vi "Process Projects.vi"(7 "Total Memory":T1, 8 "error in (no error)":errorcluster {"code" format="Error %.0f"}, 10 "Projects":refnum<class "Project Documentation.lvclass">[](array[class]), 11 "VIDoc Printer In":refnum<class "VIDoc Printer.lvclass">) -> (0 "error out":errorcluster {"code" format="Error %.0f"}, 3 "VIDoc Printer Out":refnum<class "VIDoc Printer.lvclass">)   [LabVIEW 2023, in "VIDoc Printer.lvlib" / "VIDoc Printer.lvclass"]
uses:
  VIDoc Printer.lvclass
  <vilib>/DMC/VIDoc/Framework/UI Interaction/Interface/UI Interaction.lvclass
  Parsing/Project Documentation/Project Documentation.lvclass
  Parsing/TypeDefs/Memory Size Cluster.ctl
  Parsing/VIDoc Parsing.lvlib
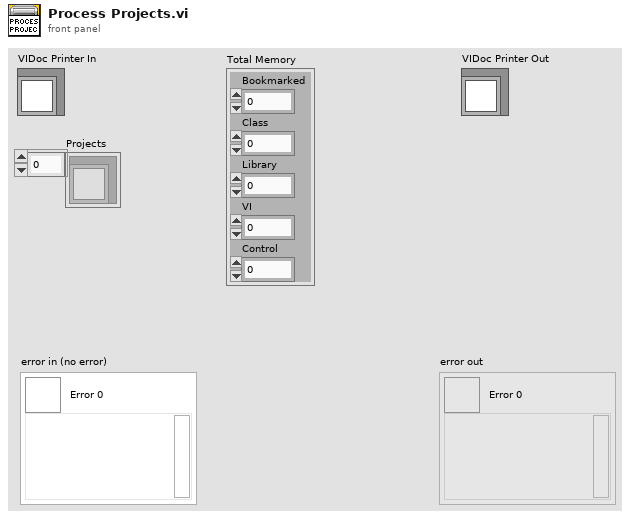
[diagram p1: front panel]
types:
  T1 = typedef "VIDoc Parsing.lvlib/Memory Size Cluster.ctl" = cluster{"Bookmarked":dbl, "Class":dbl, "Library":dbl, "VI":dbl, "Control":dbl}
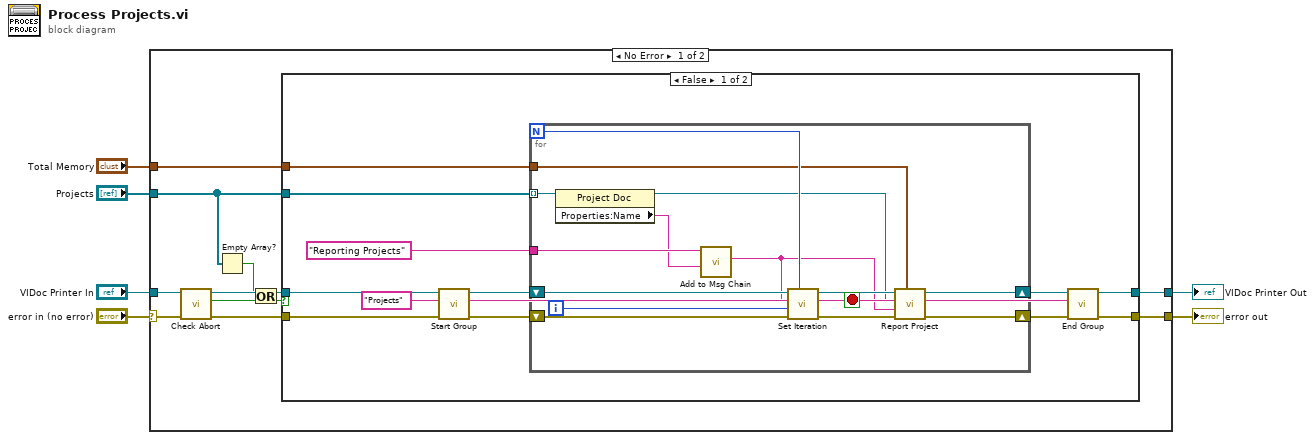
[diagram p0: block diagram]
diagram:
  n1 = case shown="No Error" "error in (no error)" {
    selector: "error in (no error)" -> [w17 w48]
    tunnel: [w12 w48] -> w5
    tunnel: [w11 w47] -> w3
    tunnel: "VIDoc Printer In" -> [w14 w47]
    tunnel: "Projects" -> [w9 _]
    tunnel: "Total Memory" -> [w10 _]
    frame No Error {
      n2 = call "Check Abort.vi"("error in (no error)"=w17, "VIDoc Printer In"=w14) -> ("error out"=w16:errorcluster, "Abort?"=w13:bool, "VIDoc Printer Out"=w15:refnum<class "VIDoc Printer.lvclass">)  [unwired: 7 in]
      n3 = Empty Array?(array=w9) -> (empty?=w7:bool)
      n4 = Or(x=w7, y=w13) -> (x .or. y?=w8:bool)
      n5 = case shown="False" w8 {
        tunnel: w9 -> [w27 _]
        tunnel: w16 -> [w26 w46]
        tunnel: w15 -> [w25 w45]
        tunnel: [w21 w46] -> w12
        tunnel: [w23 w45] -> w11
        tunnel: w10 -> [w19 _]
        frame False {
          w18 = "Projects" ("Section")
          n6 = call-dynamic "Start Group.vi"("error in (no error)"=w26, "Group"=w18, "VIDoc Printer In"=w25) -> ("error out"=w28:errorcluster, "VIDoc Printer Out"=w29:refnum<class "VIDoc Printer.lvclass">)  [unwired: 7 in]
          n7 = for {
            N -> [w38]
            shift-right: [w44] -> w24
            shift-left: w29 -> [w42]
            shift-right: [w43] -> w22
            shift-left: w28 -> [w40]
            tunnel: w27 -> [w36] mode=indexing
            tunnel: "Reporting Projects" ("Section") -> [w32]
            tunnel: w19 -> [w33]
            i -> [w37]
            stop <- w35 stop-if-true
            n8 = property class="Project Doc"(reference=w36) -> (reference out=w34:refnum<class "Project Documentation.lvclass">, "Properties:Name"=w31:string)  [unwired: 1 in, 1 out]
            n9 = call <vilib>:"Add to Msg Chain.vi"("New"=w31, "Msg Chain in"=w32) -> ("Msg Chain out"=w30:string)  [unwired: 9 in]
            n10 = call "Set Iteration.vi"("Progress Max"=w38, "error in (no error)"=w40, "Progress Value"=w37, "Message (No Message Update)"=w30, "VIDoc Printer In"=w42) -> ("error out"=w39:errorcluster, "Abort?"=w35:bool, "VIDoc Printer Out"=w41:refnum<class "VIDoc Printer.lvclass">)  [unwired: 4 in]
            n11 = call-dynamic "Report Project.vi"("Memory"=w33, "error in (no error)"=w39, "Msg Chain"=w30, "Project Doc"=w34, "VIDoc Printer In"=w41) -> ("error out"=w43:errorcluster, "VIDoc Printer Out"=w44:refnum<class "VIDoc Printer.lvclass">)  [unwired: 5 in]
          }
          n12 = call-dynamic "End Group.vi"("error in (no error)"=w22, "Group"=w18, "VIDoc Printer In"=w24) -> ("error out"=w21:errorcluster, "VIDoc Printer Out"=w23:refnum<class "VIDoc Printer.lvclass">)  [unwired: 7 in]
        }
        frame True {
        }
      }
    }
    frame Error {
    }
  }
  "error out" <- w5
  "VIDoc Printer Out" <- w3
